vi "OverVolateMessage.vi"() -> ()   [LabVIEW 2016]
panel:
  out "Message":string="OverVolatge"
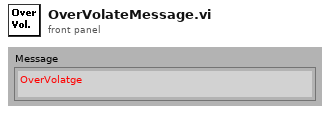
[diagram p1: front panel]
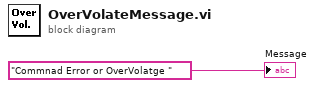
[diagram p0: block diagram]
diagram:
  "Message" <- "Commnad Error or OverVolatge "
